vi "Tree_Edit_GBD.vi"(4 "MODE":string, 6 "TAG":string, 9 "File":string[][](array[string]), 10 "Folder":string[](array[string]), 11 "Tree":refnum<vi>) -> (3 "Tree.Ref":refnum<vi>)   [LabVIEW 2017]
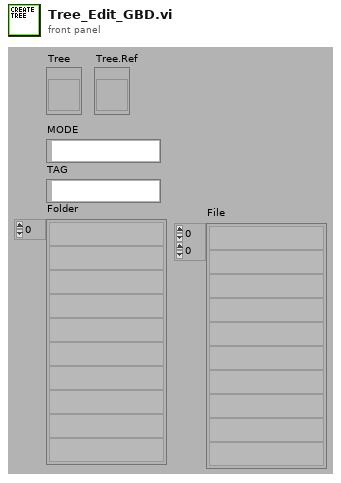
[diagram p1: front panel]
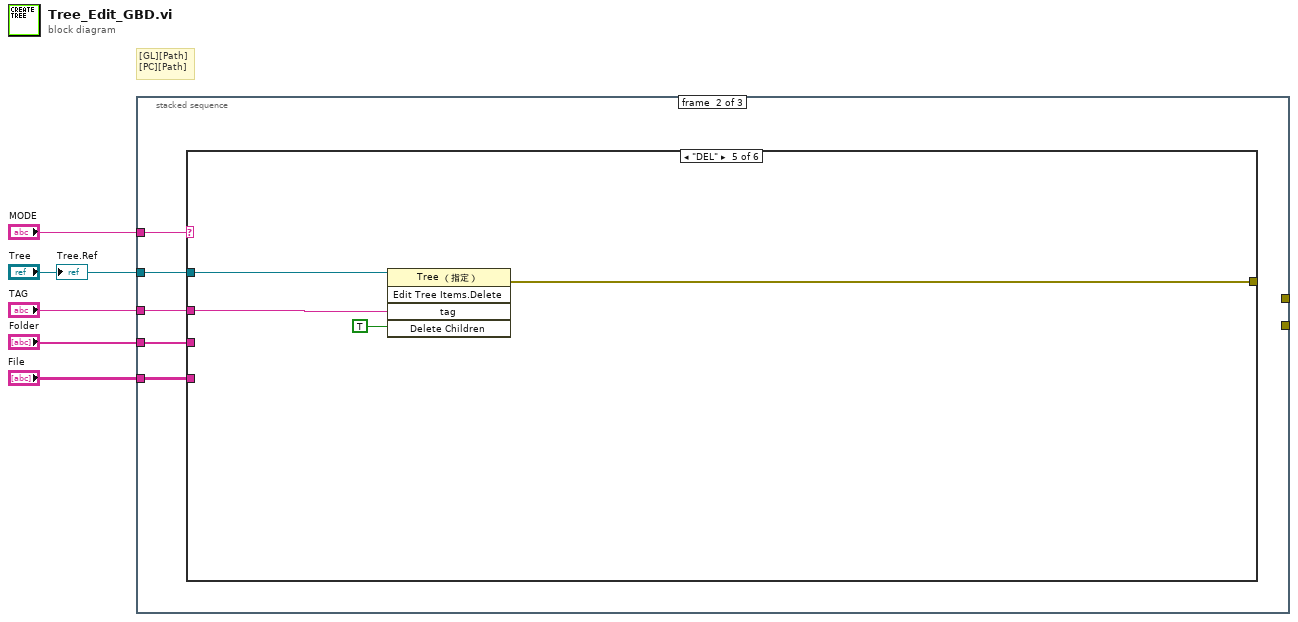
[diagram p0: block diagram]
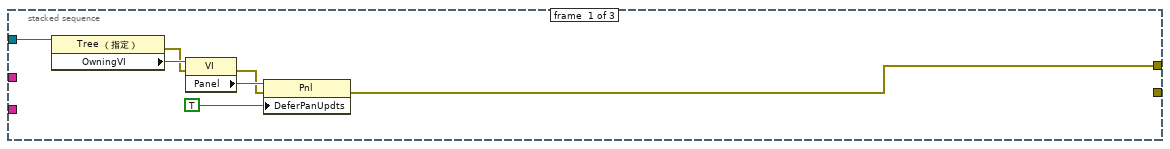
[diagram p2: hidden frame]
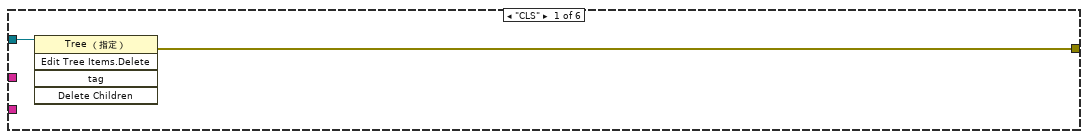
[diagram p3: hidden frame]
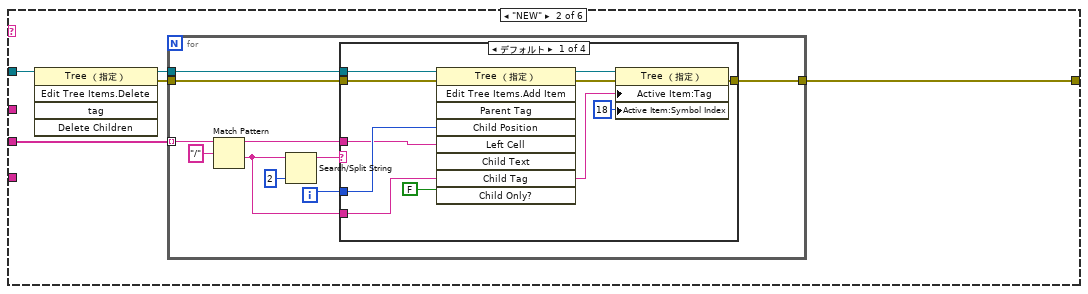
[diagram p4: hidden frame]
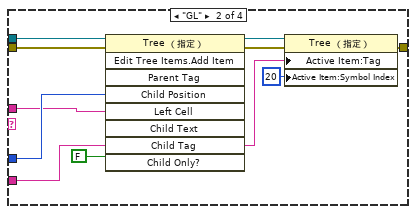
[diagram p5: hidden frame]
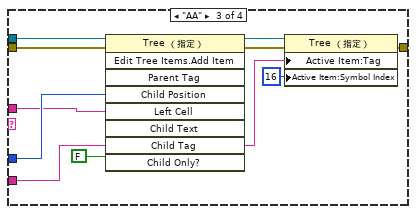
[diagram p6: hidden frame]
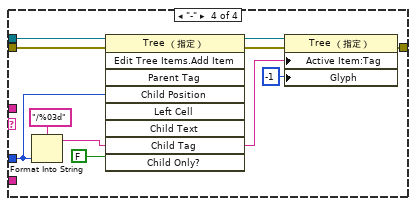
[diagram p7: hidden frame]
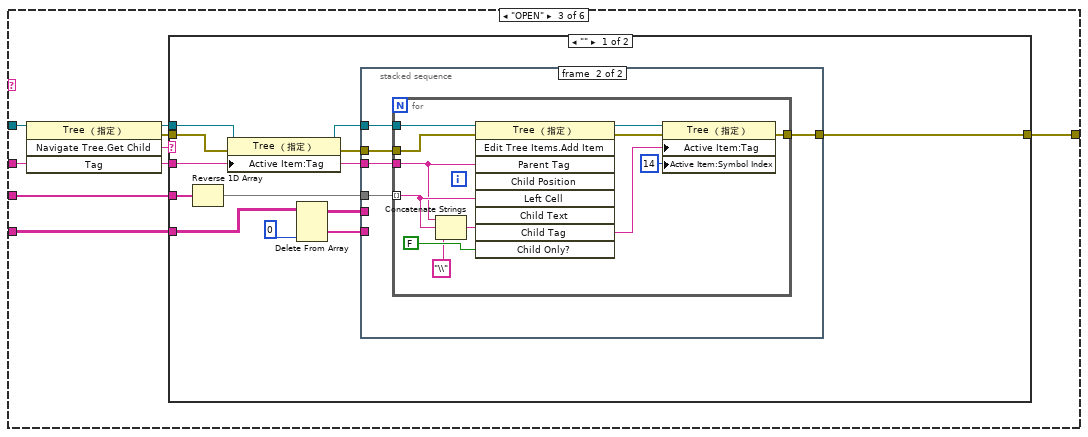
[diagram p8: hidden frame]
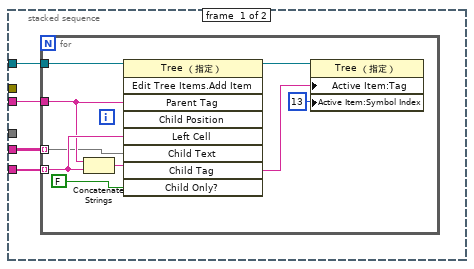
[diagram p9: hidden frame]
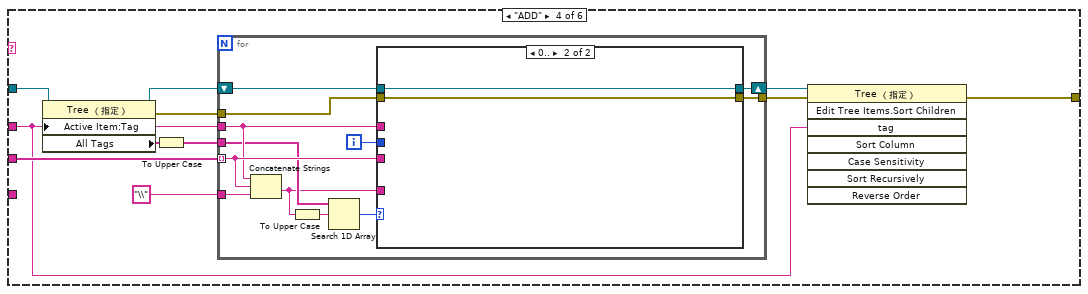
[diagram p11: hidden frame]
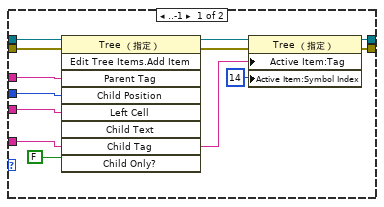
[diagram p12: hidden frame]
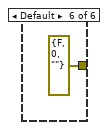
[diagram p13: hidden frame]
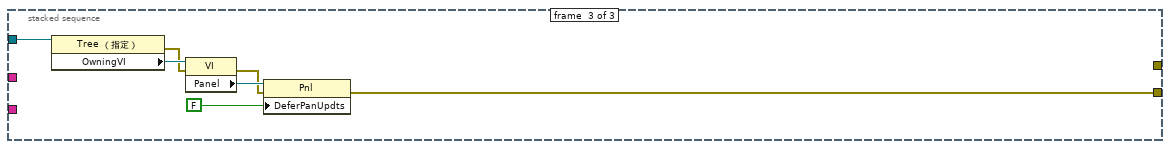
[diagram p14: hidden frame]
diagram:
  # "[GL][Path]\n[PC][Path]"
  n1 = stacked-sequence {
    tunnel: "MODE" -> [_ w17 _]
    tunnel: "Tree" -> [w12 w16 w172]
    tunnel: "TAG" -> [_ w15 _]
    tunnel: "Folder" -> [_ w14 _]
    tunnel: "File" -> [_ w13 _]
    tunnel: [_ _ w166] -> _
    tunnel: [w6 _ _] -> _
    frame #0 {
      n2 = property class="Tree （指定）"(reference=w12) -> (error out=w8:errorcluster, "OwningVI"=w11:refnum<vi>)  [unwired: 1 in, 1 out]
      n3 = property class="VI"(reference=w11, error in=w8) -> (error out=w7:errorcluster, "Panel"=w10:refnum<vi>)  [unwired: 1 out]
      n4 = property class="Pnl"(reference=w10, error in=w7, "DeferPanUpdts"=TRUE ("Defer Panel Updates")) -> (error out=w6:errorcluster)  [unwired: 1 out]
    }
    frame #1 {
      n5 = case shown="\"DEL\"" w17 {
        tunnel: w16 -> [w19 w24 w81 w131 w164 _]
        tunnel: w15 -> [_ _ w78 w129 w163 _]
        tunnel: w14 -> [_ w22 w79 w134 _ _]
        tunnel: w13 -> [_ _ w77 _ _ _]
        tunnel: [w18 w21 w75 w126 w162 errorcluster {"status"=FALSE, "code"=0, "source"=""} ("error out")] -> _
        frame "CLS" {
          n6 = invoke on="Invoke Node" class="Tree （指定）" method="Edit Tree Items.Delete"(reference=w19) -> (error out=w18:errorcluster)  [unwired: 4 in, 4 out]
        }
        frame "NEW" {
          n7 = invoke on="Invoke Node" class="Tree （指定）" method="Edit Tree Items.Delete"(reference=w24) -> (reference out=w23:refnum<vi>, error out=w20:errorcluster)  [unwired: 4 in, 3 out]
          n8 = for {
            tunnel: w23 -> [w34]
            tunnel: w22 -> [w29] mode=indexing
            tunnel: [w26] -> w21
            tunnel: w20 -> [w25]
            i -> [w33]
            n9 = Match Pattern(string=w29, regular expression="/") -> (before substring=w31:string, after substring=w27:string)  [unwired: 3 out]
            n10 = Search/Split String(string=w27, offset (0)=2) -> (substring before match=w28:string)  [unwired: 3 out]
            n11 = case shown="デフォルト" w28 {
              tunnel: w34 -> [w44 w54 w64 w74]
              tunnel: w33 -> [w40 w50 w60 w69]
              tunnel: w31 -> [w39 w49 w59 _]
              tunnel: w27 -> [w38 w48 w58 _]
              tunnel: [w37 w47 w57 w65] -> w26
              tunnel: w25 -> [w35 w45 w55 w67]
              frame Default {
                n12 = invoke on="Invoke Node" class="Tree （指定）" method="Edit Tree Items.Add Item"(reference=w44, error in=w35, "Child Position"=w40, "Left Cell"=w39, "Child Tag"=w38, "Child Only?"=FALSE) -> (reference out=w43:refnum<vi>, error out=w36:errorcluster)  [unwired: 3 in, 7 out]
                n13 = property class="Tree （指定）"(reference=w43, error in=w36, "Active Item:Tag"=w38, "Active Item:Symbol Index"=18 ("Active Item Properties:Symbol Index")) -> (error out=w37:errorcluster)  [unwired: 1 out]
              }
              frame "GL" {
                n14 = invoke on="Invoke Node" class="Tree （指定）" method="Edit Tree Items.Add Item"(reference=w54, error in=w45, "Child Position"=w50, "Left Cell"=w49, "Child Tag"=w48, "Child Only?"=FALSE) -> (reference out=w53:refnum<vi>, error out=w46:errorcluster)  [unwired: 3 in, 7 out]
                n15 = property class="Tree （指定）"(reference=w53, error in=w46, "Active Item:Tag"=w48, "Active Item:Symbol Index"=20 ("Active Item Properties:Symbol Index")) -> (error out=w47:errorcluster)  [unwired: 1 out]
              }
              frame "AA" {
                n16 = invoke on="Invoke Node" class="Tree （指定）" method="Edit Tree Items.Add Item"(reference=w64, error in=w55, "Child Position"=w60, "Left Cell"=w59, "Child Tag"=w58, "Child Only?"=FALSE) -> (reference out=w63:refnum<vi>, error out=w56:errorcluster)  [unwired: 3 in, 7 out]
                n17 = property class="Tree （指定）"(reference=w63, error in=w56, "Active Item:Tag"=w58, "Active Item:Symbol Index"=16 ("Active Item Properties:Symbol Index")) -> (error out=w57:errorcluster)  [unwired: 1 out]
              }
              frame "-" {
                n18 = Format Into String(format string="/%03d", w69) -> (resulting string=w70:string)  [unwired: 2 in, 1 out]
                n19 = invoke on="Invoke Node" class="Tree （指定）" method="Edit Tree Items.Add Item"(reference=w74, error in=w67, "Child Position"=w69, "Child Tag"=w70, "Child Only?"=FALSE) -> (reference out=w73:refnum<vi>, error out=w66:errorcluster)  [unwired: 4 in, 7 out]
                n20 = property class="Tree （指定）"(reference=w73, error in=w66, "Active Item:Tag"=w70, "Glyph"=-1 ("Active Item:Symbol Index")) -> (error out=w65:errorcluster)  [unwired: 1 out]
              }
            }
          }
        }
        frame "OPEN" {
          n21 = invoke on="Invoke Node" class="Tree （指定）" method="Navigate Tree.Get Child"(reference=w81, "Tag"=w78) -> (reference out=w82:refnum<vi>, error out=w76:errorcluster, "Navigate Tree:Get Child"=w80:string)  [unwired: 2 in, 1 out]
          n22 = case shown="\"\"" w80 {
            tunnel: w82 -> [w94 _]
            tunnel: w78 -> [w93 _]
            tunnel: w79 -> [w87 _]
            tunnel: w77 -> [w91 _]
            tunnel: w76 -> [w84 w123]
            tunnel: [w83 w123] -> w75
            frame "" {
              n23 = Reverse 1D Array(array=w87) -> (reversed array=w86:string[])
              n24 = property class="Tree （指定）"(reference=w94, error in=w84, "Active Item:Tag"=w93) -> (reference out=w92:refnum<vi>, error out=w85:errorcluster)
              n25 = Delete From Array(array=w91, index (col)=0 ("index (row)")) -> (deleted portion=w90:string[], array with subset deleted=w89:string[][])  [unwired: 2 in]
              n26 = stacked-sequence {
                tunnel: w93 -> [w98 w111]
                tunnel: w86 -> [_ w110]
                tunnel: w92 -> [w96 w109]
                tunnel: w90 -> [w97 _]
                tunnel: w89 -> [w95 _]
                tunnel: w85 -> [_ w108]
                tunnel: [_ w107] -> w83
                frame #0 {
                  n27 = for {
                    tunnel: w97 -> [w103] mode=indexing
                    tunnel: w98 -> [w102]
                    tunnel: w96 -> [w101]
                    tunnel: w95 -> [w100] mode=indexing
                    n28 = Concatenate Strings(w102, w103) -> (w99:string)
                    n29 = invoke on="Invoke Node" class="Tree （指定）" method="Edit Tree Items.Add Item"(reference=w101, "Parent Tag"=w102, "Left Cell"=w103, "Child Text"=w100, "Child Tag"=w99, "Child Only?"=FALSE) -> (reference out=w106:refnum<vi>)  [unwired: 3 in, 8 out]
                    n30 = property class="Tree （指定）"(reference=w106, "Active Item:Tag"=w99, "Active Item:Symbol Index"=13 ("Active Item Properties:Symbol Index")) -> ()  [unwired: 1 in, 2 out]
                  }
                }
                frame #1 {
                  n31 = for {
                    tunnel: w110 -> [w119] mode=indexing
                    tunnel: w111 -> [w117]
                    tunnel: w109 -> [w116]
                    tunnel: w108 -> [w113]
                    tunnel: [w112] -> w107
                    n32 = Concatenate Strings(w117, w119, "\\" ("string")) -> (w118:string)
                    n33 = invoke on="Invoke Node" class="Tree （指定）" method="Edit Tree Items.Add Item"(reference=w116, error in=w113, "Parent Tag"=w117, "Left Cell"=w119, "Child Tag"=w118, "Child Only?"=FALSE) -> (reference out=w122:refnum<vi>, error out=w114:errorcluster)  [unwired: 3 in, 7 out]
                    n34 = property class="Tree （指定）"(reference=w122, error in=w114, "Active Item:Tag"=w118, "Active Item:Symbol Index"=14 ("Active Item Properties:Symbol Index")) -> (error out=w112:errorcluster)  [unwired: 1 out]
                  }
                }
              }
            }
            frame Default {
            }
          }
        }
        frame "ADD" {
          n35 = property class="Tree （指定）"(reference=w131, "Active Item:Tag"=w129) -> (reference out=w132:refnum<vi>, error out=w125:errorcluster, "All Tags"=w128:string[])  [unwired: 1 in]
          n36 = To Upper Case(1:w128) -> (0:w127:string[])
          n37 = for {
            tunnel: w134 -> [w145] mode=indexing
            tunnel: w129 -> [w144]
            tunnel: "\\" -> [w142]
            shift-right: [w141] -> w130
            shift-left: w132 -> [w146]
            tunnel: w127 -> [w140]
            tunnel: w125 -> [w136]
            tunnel: [w135] -> w124
            i -> [w143]
            n38 = Concatenate Strings(w144, w145, w142) -> (w139:string)
            n39 = To Upper Case(1:w139) -> (0:w137:string)
            n40 = Search 1D Array(1D array=w140, element=w137) -> (index of element=w138:i32)  [unwired: 1 out]
            n41 = case shown="0.." w138 {
              tunnel: w146 -> [w158 w160]
              tunnel: w145 -> [w154 _]
              tunnel: w144 -> [w153 _]
              tunnel: w143 -> [w152 _]
              tunnel: [w151 w160] -> w141
              tunnel: w139 -> [w150 _]
              tunnel: w136 -> [w149 w159]
              tunnel: [w147 w159] -> w135
              frame ..-1 {
                n42 = invoke on="Invoke Node" class="Tree （指定）" method="Edit Tree Items.Add Item"(reference=w158, error in=w149, "Parent Tag"=w153, "Child Position"=w152, "Left Cell"=w154, "Child Tag"=w150, "Child Only?"=FALSE) -> (reference out=w157:refnum<vi>, error out=w148:errorcluster)  [unwired: 2 in, 7 out]
                n43 = property class="Tree （指定）"(reference=w157, error in=w148, "Active Item:Tag"=w150, "Active Item:Symbol Index"=14 ("Active Item Properties:Symbol Index")) -> (reference out=w151:refnum<vi>, error out=w147:errorcluster)
              }
              frame 0.. {
              }
            }
          }
          n44 = invoke on="Invoke Node" class="Tree （指定）" method="Edit Tree Items.Sort Children"(reference=w130, error in=w124, "tag"=w129) -> (error out=w126:errorcluster)  [unwired: 5 in, 7 out]
        }
        frame "DEL" {
          n45 = invoke on="Invoke Node" class="Tree （指定）" method="Edit Tree Items.Delete"(reference=w164, "tag"=w163, "Delete Children"=TRUE ("Delete Children?")) -> (error out=w162:errorcluster)  [unwired: 2 in, 4 out]
        }
        frame Default {
        }
      }
    }
    frame #2 {
      n46 = property class="Tree （指定）"(reference=w172) -> (error out=w168:errorcluster, "OwningVI"=w171:refnum<vi>)  [unwired: 1 in, 1 out]
      n47 = property class="VI"(reference=w171, error in=w168) -> (error out=w167:errorcluster, "Panel"=w170:refnum<vi>)  [unwired: 1 out]
      n48 = property class="Pnl"(reference=w170, error in=w167, "DeferPanUpdts"=FALSE ("Defer Panel Updates")) -> (error out=w166:errorcluster)  [unwired: 1 out]
    }
  }
  "Tree.Ref" <- "Tree"
